vi "hari 1.vi"() -> ()   [LabVIEW 2020]
panel:
  out "array of clusters":cluster{string, string, string}[](array[cluster])
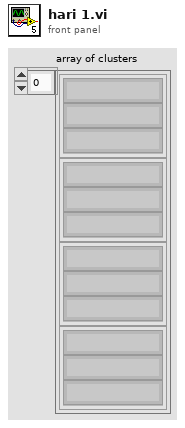
[diagram p1: front panel]
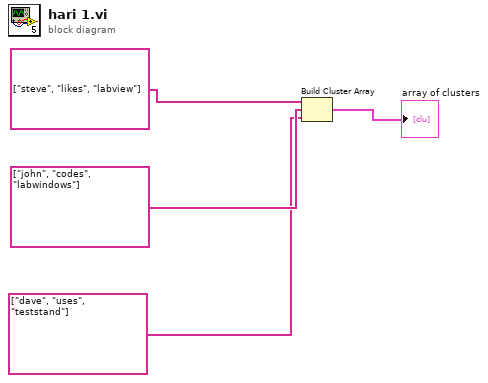
[diagram p0: block diagram]
diagram:
  n1 = Build Cluster Array(string[] ["steve", "likes", "labview"], string[] ["john", "codes", "labwindows"], string[] ["dave", "uses", "teststand"]) -> (→"array of clusters":cluster{string, string, string}[])
